vi "Scalar JSON text to Variant.vi"(6 "Type":T1, 8 "error in (no error)":errorcluster, 9 "Variant (Data Type)":variant, 10 "Offset":i32, 11 "JSON":string) -> (0 "error out":errorcluster, 1 "Variant out":variant)   [LabVIEW 2020, in "JSONtext.lvlib"]
uses:
  <vilib>/JDP Science/JSONtext/JSONtext.lvlib
  <vilib>/Utility/Data Type/Type Definitions/Data Type.ctl
  <vilib>/Utility/Data Type/Type Definitions/Refnum Type.ctl
  <vilib>/JDP Science/JSONtext/Parsing/Advance past String.vi
  <vilib>/JDP Science/JSONtext/String Subset.vi
  <vilib>/JDP Science/JSONtext/support/Strip Quotes and Unescape.vi
  <vilib>/JDP Science/JSONtext/support/Get Number Text.vi
  <vilib>/JDP Science/JSONtext/Parsing/NaN or null to Integer ERROR.vi
  <vilib>/JDP Science/JSONtext/Parsing/Advance past Number.vi
  <vilib>/JDP Science/JSONtext/Parsing/Advance past Line Ending.vi
  <vilib>/JDP Science/JSONtext/support/Unescape JSON string.vi
  <vilib>/JDP Science/JSONtext/Parsing/Parsing Error in converting to LabVIEW type.vi
  <vilib>/JDP Science/JDP Science Common Utilities/Timestamp/Text to Timestamp.vi
  <vilib>/Utility/Data Type/NI_Data Type.lvlib
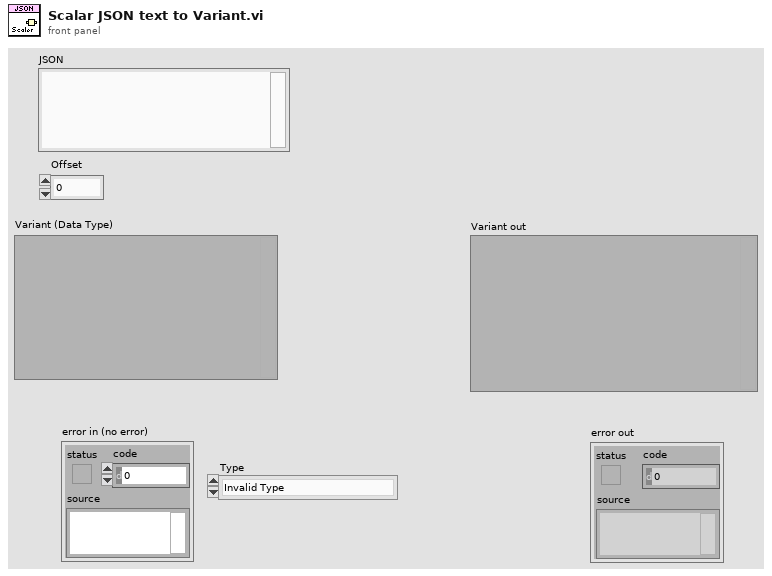
[diagram p1: front panel]
types:
  T1 = typedef "NI_Data Type.lvlib/Data Type.ctl" = enum8{"Invalid Type", "Void", "I8", "I16", "I32", "I64", "U8", "U16", "U32", "U64", "Single Float", "Double Float", "Extended Float", "Single Complex", "Double Complex", "Extended Complex", "Enum U8", "Enum U16", "Enum U32", "Enum U64", "Single Float With Unit", "Double Float With Unit", "Extended Float With Unit", "Single Complex with Unit", "Double Complex with Unit", "Extended Complex with Unit", "Boolean", "String", "Path", "Picture", "Tag", "Array", "Cluster", "Variant", "LV Variant", "Waveform", "Timestamp", "Digital Waveform", "Digital Data", "ExpressData", "Refnum", "External Data", "VI", "Poly VI", "LabVIEW Class Instance", "Fixed Point", "Set Collection", "Map Collection"}
  T2 = typedef "JSONtext.lvlib/Parsing State.ctl" = enum16{"Parser Error", "Object", "Array", "String", "Number/Other", "Leading Whitespace", "Object end", "Array end", "Value end"}
  T3 = typedef "NI_Data Type.lvlib/Refnum Type.ctl" = enum16{"NotARefnum", "UnknownRefnum", "Generic", "Datalog", "ByteStream", "Device", "Occurence", "TCPNetConnection", "Auto", "Menu", "Imaq", "Hardware", "DataSocket", "Visa", "IVI", "UDPNetConnection", "Notifier", "Queue", "Irda", "EventReg", "DotNet", "UserEvent", "Callback", "UNUSED_EMPTY_POSITION", "BlueToothNetConnection", "LVObjApp", "LVObjVI", "LVObjUnknown", "GenericClass", "UserDefinedRefnumTag", "DataValue", "RT FIFO", "TDMS File", "PythonSessionRefnum"}
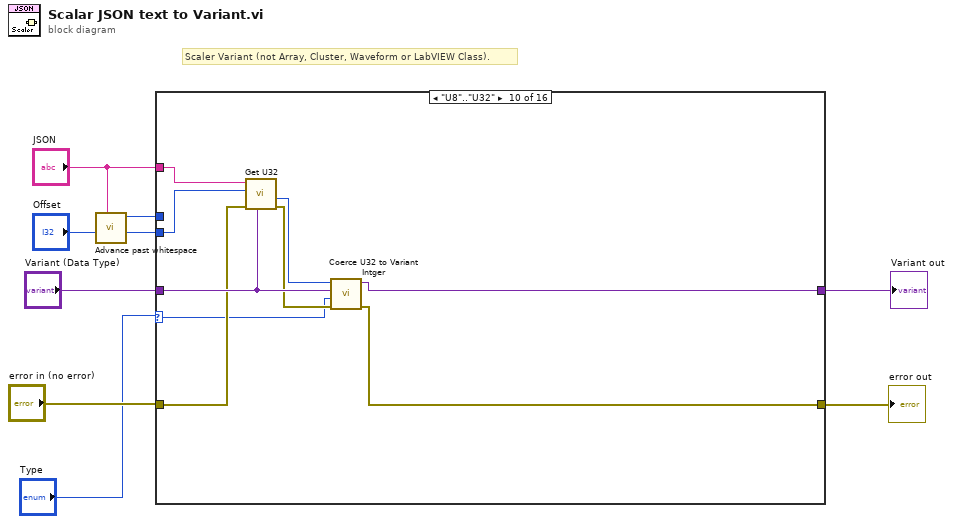
[diagram p0: block diagram]
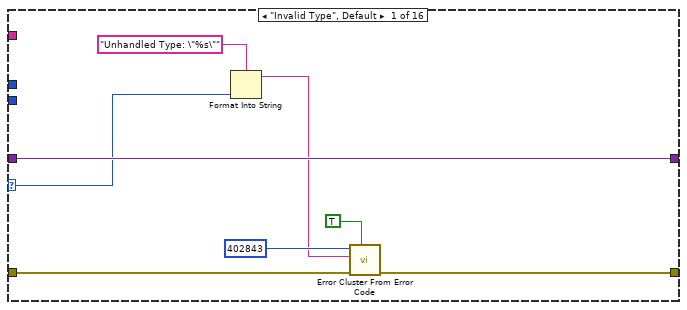
[diagram p2: hidden frame]
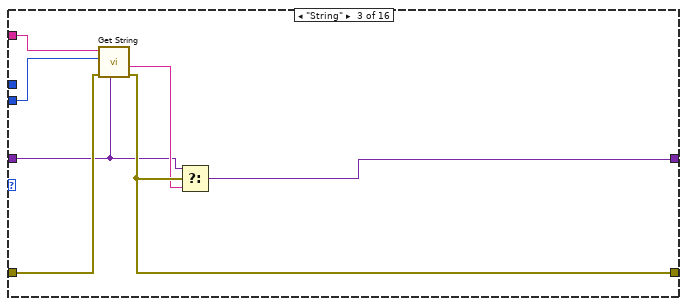
[diagram p4: hidden frame]
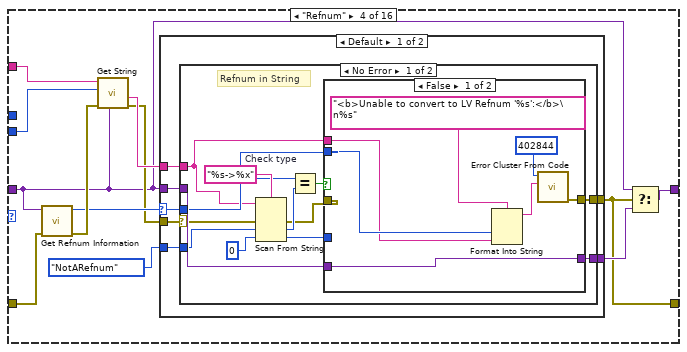
[diagram p5: hidden frame]
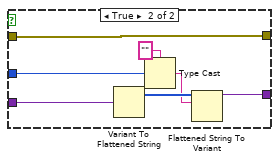
[diagram p6: hidden frame]
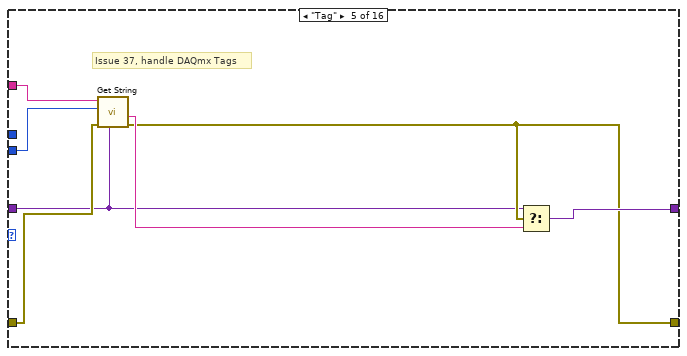
[diagram p9: hidden frame]
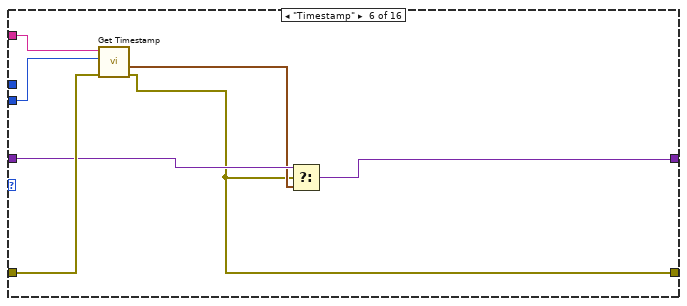
[diagram p10: hidden frame]
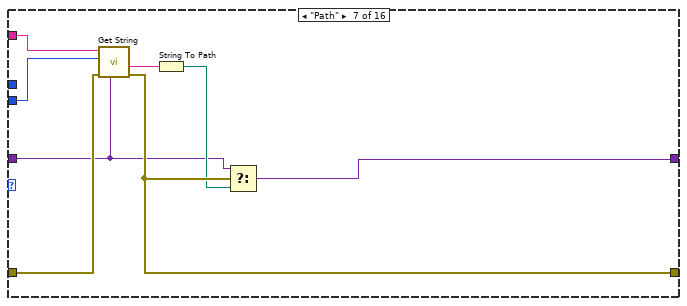
[diagram p11: hidden frame]
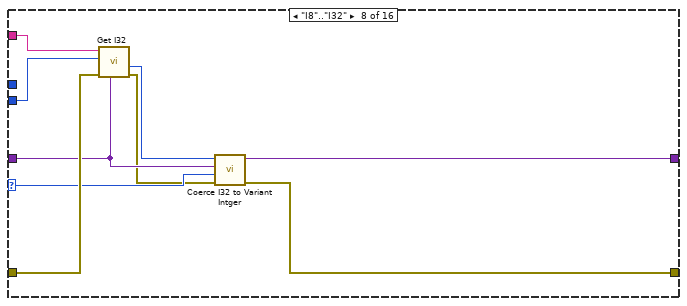
[diagram p12: hidden frame]
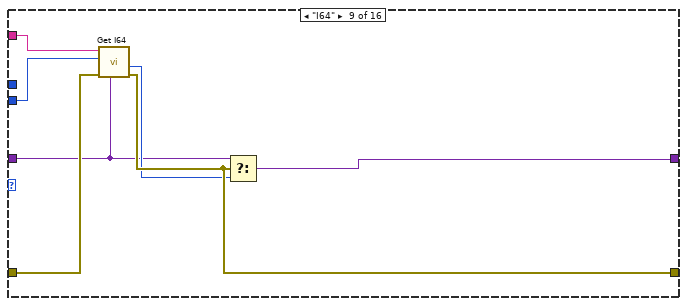
[diagram p13: hidden frame]
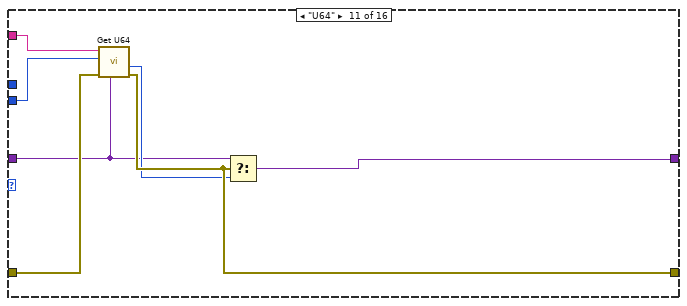
[diagram p14: hidden frame]
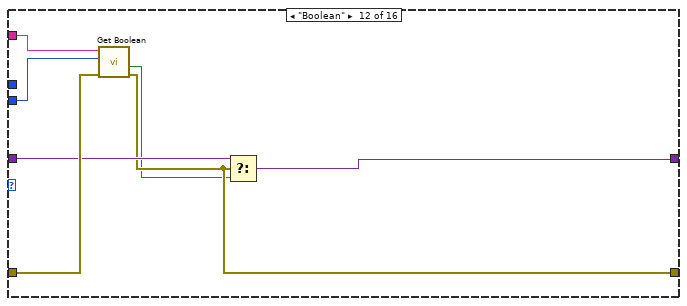
[diagram p15: hidden frame]
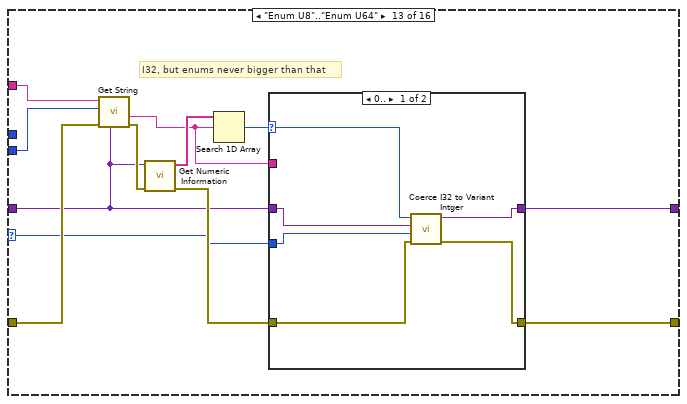
[diagram p16: hidden frame]
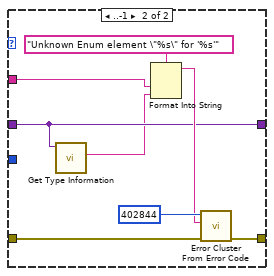
[diagram p17: hidden frame]
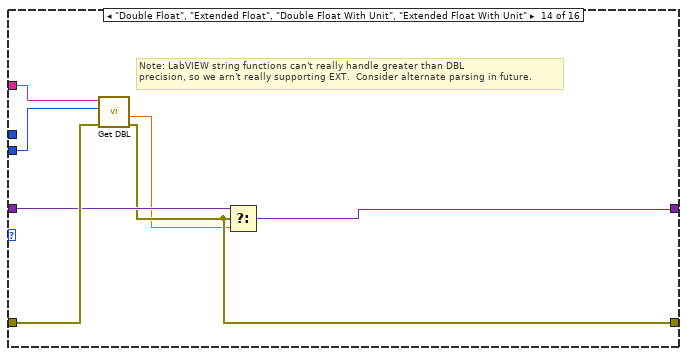
[diagram p18: hidden frame]
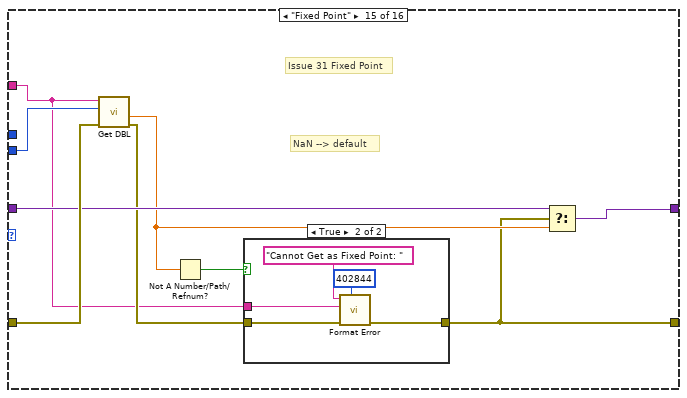
[diagram p19: hidden frame]
diagram:
  # "Scaler Variant (not Array, Cluster, Waveform or LabVIEW Class)."
  n1 = call <vilib>:"Advance past whitespace.vi"("JSON"="JSON", "Offset"="Offset") -> ("Offset of first non-whitespace"=w5:i32, "Parser State"=w3:T2)  [unwired: 7 in, 1 out]
  n2 = case shown="\"U8\"..\"U32\"" "Type" {
    selector: "Type" -> [w12 _ _ _ _ _ _ w102 _ w114 _ _ w137 _ _ _]
    tunnel: "Variant (Data Type)" -> [w16 w18 w20 w27 w76 w86 w90 w101 w107 w120 w123 w134 w138 w167 w176 w189]
    tunnel: "JSON" -> [_ _ w25 w37 w81 w88 w96 w104 w109 w121 w125 w131 w146 w164 w172 w186]
    tunnel: [w15 w19 w22 w29 w77 w83 w93 w98 w110 w117 w126 w132 w142 w165 w170 w187] -> w8
    tunnel: "error in (no error)" -> [w17 w19 w24 w35 w79 w87 w95 w105 w112 w116 w128 w135 w147 w168 w177 w190]
    tunnel: w5 -> [_ _ w26 w38 w82 w89 w97 w106 w113 w122 w129 w136 w148 w169 w178 w191]
    tunnel: [w16 w18 w23 w36 w80 w85 w94 w100 w111 w118 w127 w133 w143 w166 w175 w188] -> w7
    tunnel: w3 -> [_ _ _ _ _ _ _ _ _ _ _ _ _ _ _ _]
    frame "Invalid Type", Default {
      n3 = Format Into String(format string="Unhandled Type: \"%s\"", w12) -> (resulting string=w10:string)  [unwired: 2 in, 1 out]
      n4 = call <vilib>:"Error Cluster From Error Code.vi"("show call chain? (False)"=TRUE, "error in (no error)"=w17, "error message (\"\")"=w10, "error code (0)"=402843) -> ("error out"=w15:errorcluster)  [unwired: 5 in]
    }
    frame "Void" {
      # "Empty Variant: #ToDo Variant Attributes?"
    }
    frame "String" {
      n5 = call <vilib>:"Get String.vi"("LV Type"=w20, "error in (no error)"=w24, "Offset"=w26, "JSON"=w25) -> ("error out"=w22:errorcluster, "String"=w21:string)  [unwired: 5 in, 1 out]
      n6 = Select(t=w20, s=w22, f=w21) -> (s? t:f=w23:variant)
    }
    frame "Refnum" {
      n7 = call <vilib>:"Get Refnum Information.vi"("error in (no error)"=w35, "variant"=w27) -> ("error out"=w34:errorcluster, "reference type"=w33:T3)  [unwired: 6 in, 2 out]
      n8 = call <vilib>:"Get String.vi"("LV Type"=w27, "error in (no error)"=w34, "Offset"=w38, "JSON"=w37) -> ("error out"=w30:errorcluster, "String"=w31:string)  [unwired: 5 in, 1 out]
      n9 = case shown="Default" w33 {
        selector: w33 -> [w39 _]
        tunnel: [w44 w75] -> w32
        tunnel: w31 -> [w41 w75]
        tunnel: w27 -> [w45 _]
        tunnel: w30 -> [w43 w74]
        tunnel: [w42 w74] -> w29
        tunnel: Refnum_Type."NotARefnum" ("Reference Type") -> [w40 _]
        frame Default {
          n10 = case shown="No Error" w43 {
            selector: w43 -> [w53 w73]
            tunnel: w45 -> [w58 _]
            tunnel: [w57 _] -> w44
            tunnel: [w48 w73] -> w42
            tunnel: w41 -> [w46 _]
            tunnel: w40 -> [w52 _]
            tunnel: w39 -> [w47 _]
            frame No Error {
              # "Refnum in String"
              n11 = Scan From String(format string="%s->%x", input string=w46, error in=w53, default 1=w52, default 2=u32 0) -> (error out=w49:errorcluster, output 1=w51:T3, output 2=w54:u32)  [unwired: 1 in, 2 out]
              n12 = Equal? "Check type"(x=w47, y=w51) -> (x = y?=w50:bool)
              n13 = case shown="False" w50 {
                tunnel: w58 -> [w65 w70]
                tunnel: [w65 w69] -> w57
                tunnel: w54 -> [_ w67]
                tunnel: w49 -> [_ w66]
                tunnel: [w64 w66] -> w48
                tunnel: w47 -> [w60 _]
                tunnel: w46 -> [w59 _]
                frame False {
                  n14 = Format Into String(format string="<b>Unable to convert to LV Refnum '%s':</b>\n%s", w60, w59) -> (resulting string=w62:string)  [unwired: 2 in, 1 out]
                  n15 = call <vilib>:"Error Cluster From Code.vi"("error message (\"\")"=w62, "error code (402840+)"=402844) -> ("error out"=w64:errorcluster)  [unwired: 7 in]
                }
                frame True {
                  n16 = Variant To Flattened String(Variant=w70) -> (1:w72:i16[])  [unwired: 1 out]
                  n17 = Type Cast(type="", x=w67) -> (*(type *) &x=w71:string)
                  n18 = Flattened String To Variant(6:w71, 7:w72) -> (3:w69:variant)  [unwired: 1 in, 1 out]
                }
              }
            }
            frame Error {
            }
          }
        }
        frame "Visa", "IVI", "UserDefinedRefnumTag" {
        }
      }
      n19 = Select(t=w27, s=w29, f=w32) -> (s? t:f=w36:variant)
    }
    frame "Tag" {
      # "Issue 37, handle DAQmx Tags"
      n20 = call <vilib>:"Get String.vi"("LV Type"=w76, "error in (no error)"=w79, "Offset"=w82, "JSON"=w81) -> ("error out"=w77:errorcluster, "String"=w78:string)  [unwired: 5 in, 1 out]
      n21 = Select(t=w76, s=w77, f=w78) -> (s? t:f=w80:variant)
    }
    frame "Timestamp" {
      n22 = call <vilib>:"Get Timestamp.vi"("error in (no error)"=w87, "Offset"=w89, "JSON"=w88) -> ("error out"=w83:errorcluster, "Timestamp"=w84:timestamp)  [unwired: 6 in, 1 out]
      n23 = Select(t=w86, s=w83, f=w84) -> (s? t:f=w85:variant)
    }
    frame "Path" {
      n24 = call <vilib>:"Get String.vi"("LV Type"=w90, "error in (no error)"=w95, "Offset"=w97, "JSON"=w96) -> ("error out"=w93:errorcluster, "String"=w91:string)  [unwired: 5 in, 1 out]
      n25 = String To Path(string=w91) -> (path=w92:path)
      n26 = Select(t=w90, s=w93, f=w92) -> (s? t:f=w94:variant)
    }
    frame "I8".."I32" {
      n27 = call <vilib>:"Get I32.vi"("LV Type"=w101, "error in (no error)"=w105, "Offset"=w106, "JSON"=w104) -> ("error out"=w99:errorcluster, "Number"=w103:i32)  [unwired: 5 in, 1 out]
      n28 = call <vilib>:"Coerce I32 to Variant Intger.vi"("error in (no error)"=w99, "Type"=w102, "Default in"=w101, "I32"=w103) -> ("error out"=w98:errorcluster, "Variant (Data Type) out"=w100:variant)  [unwired: 6 in]
    }
    frame "I64" {
      n29 = call <vilib>:"Get I64.vi"("LV Type"=w107, "error in (no error)"=w112, "Offset"=w113, "JSON"=w109) -> ("error out"=w110:errorcluster, "Number"=w108:i64)  [unwired: 5 in, 1 out]
      n30 = Select(t=w107, s=w110, f=w108) -> (s? t:f=w111:variant)
    }
    frame "U8".."U32" {
      n31 = call <vilib>:"Get U32.vi"("LV Type"=w120, "error in (no error)"=w116, "Offset"=w122, "JSON"=w121) -> ("error out"=w115:errorcluster, "Number"=w119:u32)  [unwired: 5 in, 1 out]
      n32 = call <vilib>:"Coerce U32 to Variant Intger.vi"("error in (no error)"=w115, "Type"=w114, "Default in"=w120, "U32"=w119) -> ("error out"=w117:errorcluster, "Variant (Data Type) out"=w118:variant)  [unwired: 6 in]
    }
    frame "U64" {
      n33 = call <vilib>:"Get U64.vi"("LV Type"=w123, "error in (no error)"=w128, "Offset"=w129, "JSON"=w125) -> ("error out"=w126:errorcluster, "Number"=w124:u64)  [unwired: 5 in, 1 out]
      n34 = Select(t=w123, s=w126, f=w124) -> (s? t:f=w127:variant)
    }
    frame "Boolean" {
      n35 = call <vilib>:"Get Boolean.vi"("error in (no error)"=w135, "Offset"=w136, "JSON"=w131) -> ("error out"=w132:errorcluster, "Boolean"=w130:bool)  [unwired: 6 in, 1 out]
      n36 = Select(t=w134, s=w132, f=w130) -> (s? t:f=w133:variant)
    }
    frame "Enum U8".."Enum U64" {
      # "I32, but enums never bigger than that"
      n37 = call <vilib>:"Get String.vi"("LV Type"=w138, "error in (no error)"=w147, "Offset"=w148, "JSON"=w146) -> ("error out"=w140:errorcluster, "String"=w141:string)  [unwired: 5 in, 1 out]
      n38 = call <vilib>:"Get Numeric Information.vi"("error in (no error)"=w140, "variant"=w138) -> ("error out"=w139:errorcluster, "enum names"=w144:string[])  [unwired: 6 in, 2 out]
      n39 = Search 1D Array(1D array=w144, element=w141) -> (index of element=w145:i32)  [unwired: 1 in]
      n40 = case shown="0.." w145 {
        selector: w145 -> [w152 _]
        tunnel: [w151 w157] -> w143
        tunnel: w138 -> [w153 w157]
        tunnel: w139 -> [w150 w160]
        tunnel: [w149 w162] -> w142
        tunnel: w141 -> [_ w155]
        tunnel: w137 -> [w154 _]
        frame 0.. {
          n41 = call <vilib>:"Coerce I32 to Variant Intger.vi"("error in (no error)"=w150, "Type"=w154, "Default in"=w153, "I32"=w152) -> ("error out"=w149:errorcluster, "Variant (Data Type) out"=w151:variant)  [unwired: 6 in]
        }
        frame ..-1 {
          n42 = call <vilib>:"Get Type Information.vi"("variant"=w157) -> ("name"=w156:string)  [unwired: 6 in, 4 out]
          n43 = Format Into String(format string="Unknown Enum element \"%s\" for '%s'", w155, w156) -> (resulting string=w158:string)  [unwired: 2 in, 1 out]
          n44 = call <vilib>:"Error Cluster From Error Code.vi"("error in (no error)"=w160, "error message (\"\")"=w158, "error code (0)"=402844) -> ("error out"=w162:errorcluster)  [unwired: 6 in]
        }
      }
    }
    frame "Double Float", "Extended Float", "Double Float With Unit", "Extended Float With Unit" {
      # "Note: LabVIEW string functions can't really handle greater than DBL\nprecision, so we arn't really supporting EXT.  Consider alternate parsing in future."
      n45 = call <vilib>:"Get DBL.vi"("error in (no error)"=w168, "Offset"=w169, "JSON"=w164) -> ("error out"=w165:errorcluster, "Number"=w163:dbl)  [unwired: 6 in, 1 out]
      n46 = Select(t=w167, s=w165, f=w163) -> (s? t:f=w166:variant)
    }
    frame "Fixed Point" {
      # "NaN --> default"
      # "Issue 31 Fixed Point"
      n47 = call <vilib>:"Get DBL.vi"("error in (no error)"=w177, "Offset"=w178, "JSON"=w172) -> ("error out"=w173:errorcluster, "Number"=w174:dbl)  [unwired: 6 in, 1 out]
      n48 = Not A Number/Path/Refnum?(number/path/refnum=w174) -> (NaN/Path/Refnum?=w171:bool)
      n49 = case shown="True" w171 {
        tunnel: w173 -> [w179 w184]
        tunnel: [w179 w183] -> w170
        tunnel: w172 -> [_ w180]
        frame False {
        }
        frame True {
          n50 = call <vilib>:"Format Error.vi"("error code (402842)"=402844, "error in (no error)"=w184, "message part 2"=w180, "error message"="Cannot Get as Fixed Point: " ("format string")) -> ("error out"=w183:errorcluster)  [unwired: 7 in]
        }
      }
      n51 = Select(t=w176, s=w170, f=w174) -> (s? t:f=w175:variant)
    }
    frame "Single Float", "Single Float With Unit" {
      n52 = call <vilib>:"Get SGL.vi"("error in (no error)"=w190, "Offset"=w191, "JSON"=w186) -> ("error out"=w187:errorcluster, "Number"=w185:sgl)  [unwired: 6 in, 1 out]
      n53 = Select(t=w189, s=w187, f=w185) -> (s? t:f=w188:variant)
    }
  }
  "Variant out" <- w7
  "error out" <- w8
